vi "getA.vi"(10 "format string":string, 11 "format string 2":string) -> (3 "result string":string)   [LabVIEW 2017]
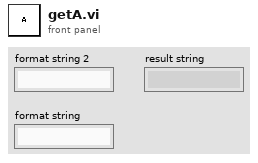
[diagram p1: front panel]
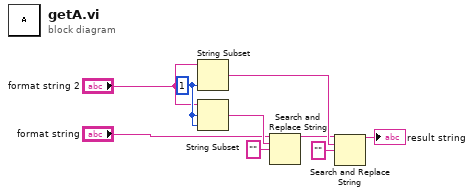
[diagram p0: block diagram]
diagram:
  w2 = 1 ("length (rest)")
  n1 = String Subset(string="format string 2", length (rest)=w2) -> (substring=w7:string)  [unwired: 1 in]
  n2 = String Subset(string="format string 2", offset (0)=w2, length (rest)=w2) -> (substring=w4:string)
  n3 = Search and Replace String(input string="format string", search string=w4, replace string="" ("replace string (\"\")")) -> (result string=w6:string)  [unwired: 5 in, 3 out]
  n4 = Search and Replace String(input string=w6, search string=w7, replace string="" ("replace string (\"\")")) -> (result string=→"result string":string)  [unwired: 5 in, 3 out]
